vi "DAQ Type Axis Scales.vi"(8 "Error In":errorcluster, 9 "Vertical Settings":T1=[{"Offset [V]"=0.5, "Coupling"=enum."DC 1 MOhm", "Range [V]"=0.0, "BW Limit"=0.0}, {"Offset [V]"=0.2, "Coupling"=enum."DC 1 MOhm", "Range [V]"=0.0, "BW Limit"=1.0}] {"BW Limit" items=["20 MHz"=20.0, "40 MHz"=40.0, "None"=-1.0]; "Range [V]" items=["0.2"=0.2, "0.4"=0.4, "1"=1.0, "2"=2.0, "4"=4.0, "10"=10.0]; "Offset [V]" format="%#_13p"}, 11 "Graph In":refnum<vi>) -> (0 "Error Out":errorcluster, 3 "Graph Out":refnum<vi>)   [LabVIEW 2019]
uses:
  NI Scope HSN/NI Scope Vertical.ctl
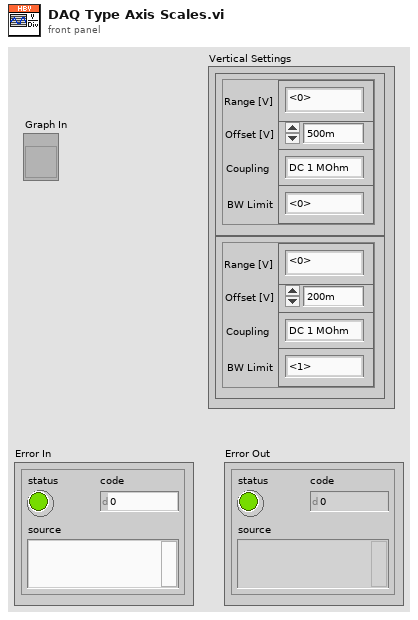
[diagram p1: front panel]
types:
  T1 = typedef "NI Scope Vertical.ctl" = cluster{"Offset [V]":dbl, "Coupling":enum16{"GND", "DC 50 Ohm", "DC 1 MOhm", "AC 1 MOhm"}, "Range [V]":dbl, "BW Limit":dbl}[]
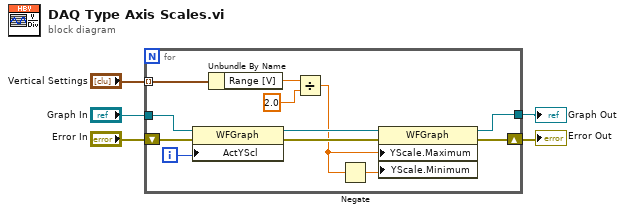
[diagram p0: block diagram]
diagram:
  n1 = for {
    shift-right: [w9] -> w5
    shift-left: "Error In" -> [w15]
    tunnel: "Vertical Settings" -> [w17] mode=indexing
    tunnel: "Graph In" -> [w14]
    tunnel: [w8] -> w2
    i -> [w13]
    n2 = property class="WFGraph"(reference=w14, error in=w15, "ActYScl"=w13) -> (reference out=w7:refnum<vi>, error out=w10:errorcluster)
    n3 = Unbundle By Name(w17) -> ("Range [V]"=w16:dbl)
    n4 = Divide(x=w16, y=2.0) -> (x/y=w6:dbl)
    n5 = Negate(x=w6) -> (-x=w11:dbl)
    n6 = property on="Property Node" class="WFGraph"(reference=w7, error in=w10, "YScale.Maximum"=w6, "YScale.Minimum"=w11) -> (reference out=w8:refnum<vi>, error out=w9:errorcluster)
  }
  "Error Out" <- w5
  "Graph Out" <- w2
